vi "Autonomous Independent.vi"() -> ()   [LabVIEW 2014]
doc: "This VI is called when autonomous begins, and will automatically be terminated when autonomous ends. You can carry out timed or sensor driven robot movement independently without needing to return to the caller."
uses:
  <vilib>/Rock Robotics/WPI/Joystick/WPI_JoystickGetSetRefNum.vi
  Support Files/Global Data!!!.vi
panel:
  out "Current State":string
  in  "Recycling Conainer?":bool
  in  "Totes Collected":i8(knob) scale=0.0..3.0
  in  "Direction?":bool
  # "Be sure to right-click and choose Data Operations>>Make Current Value default if you want to save the array values with the VI"
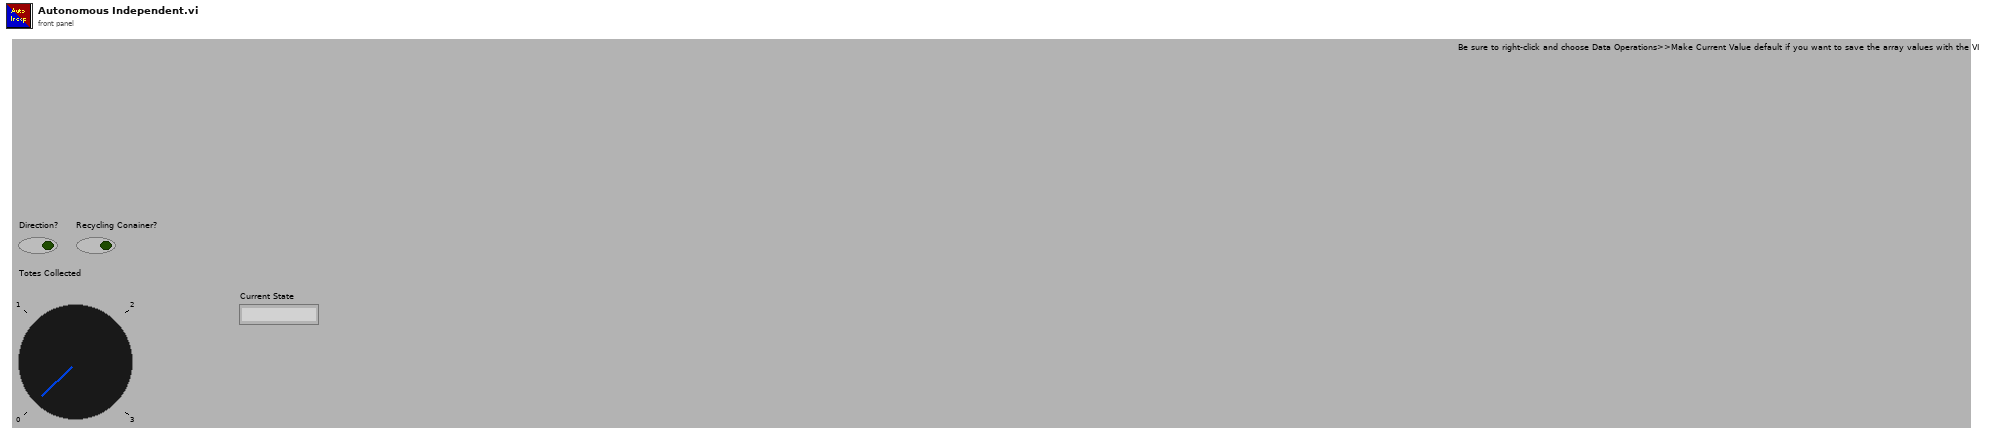
[diagram p1: front panel]
types:
  T1 = typedef "WPI_JoystickDevRef.ctl" = cluster{"Device":T2}
  T2 = typedef "WPI_JoystickDeviceEnum.ctl" = enum16{"USB 0", "USB 1", "USB 2", "USB 3", "USB 4", "USB 5"}
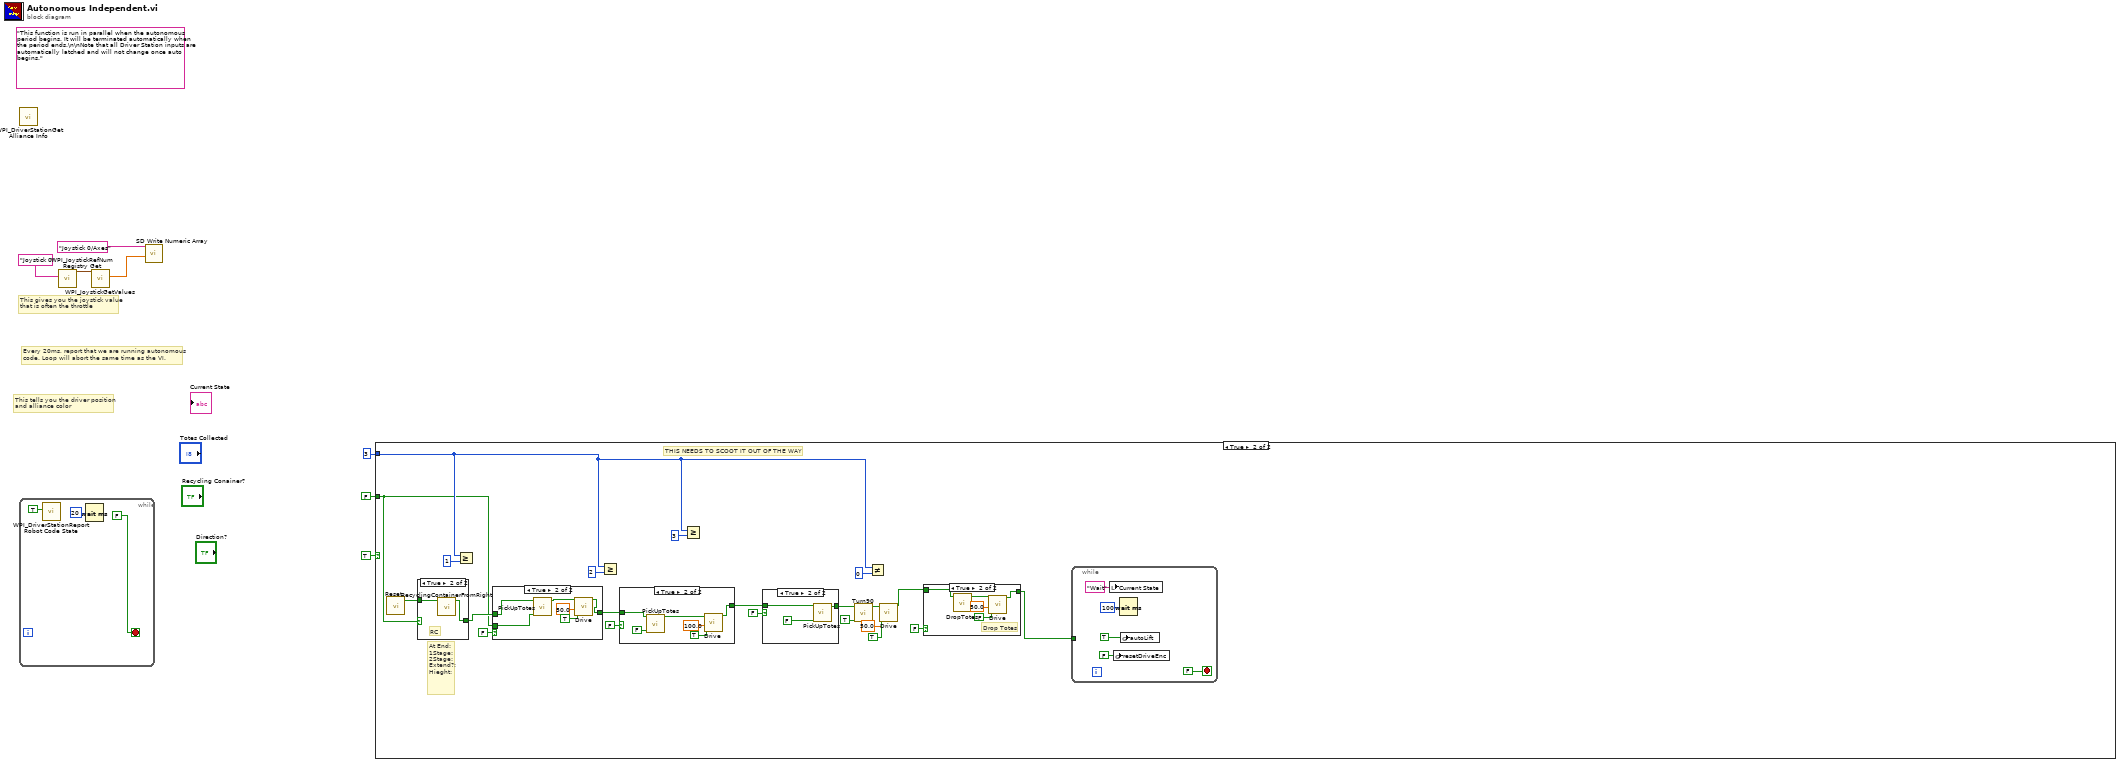
[diagram p0: block diagram]
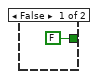
[diagram p3: hidden frame]
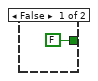
[diagram p4: hidden frame]
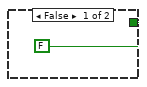
[diagram p5: hidden frame]
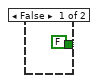
[diagram p6: hidden frame]
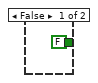
[diagram p7: hidden frame]
diagram:
  (unwired) "This function is run in parallel when the autonomous period begins. It will be terminated automatically when the period ends.\n\nNote that all Driver Station inputs are automatically latched and will not change once auto begins."
  # "Every 20ms, report that we are running autonomous\ncode. Loop will abort the same time as the VI."
  # "This gives you the joystick value\nthat is often the throttle"
  # "This tells you the driver position\nand alliance color"
  n1 = while {
    stop <- FALSE stop-if-true
    n2 = call <vilib>:"WPI_DriverStationReport Robot Code State.vi"("Autonomous"=TRUE) -> ()  [unwired: 10 in, 1 out]
    n3 = Wait (ms)(milliseconds to wait=u32 20) -> ()  [unwired: 1 out]
  }
  n4 = call <vilib>:"WPI_DriverStationGet Alliance Info.vi"() -> ()  [unwired: 12 out]
  n5 = call <vilib>:"WPI_JoystickRefNum Registry Get.vi"("refnum name"="Joystick 0") -> ("JoystickDevRef"=w6:T1)  [unwired: 1 in, 9 out]
  n6 = call <vilib>:"WPI_JoystickGetValues.vi"("JoystickDevRef"=w6) -> ("Axes"=w4:dbl[])  [unwired: 6 in, 4 out]
  n7 = call <vilib>:"SD Write Numeric Array.vi"("Numeric Array"=w4, "Name"="Joystick 0/Axes") -> ()  [unwired: 8 in, 2 out]
  n8 = case shown="True" TRUE {
    tunnel: i8 3 ("Totes Collected") -> [_ w27]
    tunnel: FALSE ("Recycling Conainer?") -> [_ w23]
    frame False {
    }
    frame True {
      # "At End:\n1Stage:\n2Stage:\nExtend?:\nHieght:"
      # "THIS NEEDS TO SCOOT IT OUT OF THE WAY"
      n9 = call "Reset.vi"() -> ("Boolean"=w24:bool)  [unwired: 11 in]
      n10 = case shown="True" w23 {
        tunnel: [FALSE w63] -> w31
        tunnel: w24 -> [_ w62]
        frame False {
        }
        frame True {
          # "RC"
          n11 = call "RecyclingContainerFromRight.vi"("Boolean In"=w62) -> ("Boolean Out"=w63:bool)  [unwired: 9 in]
        }
      }
      n12 = Greater Or Equal?(x=w27, y=i8 1) -> ()  [unwired: 1 out]
      n13 = case shown="True" FALSE {
        tunnel: w31 -> [_ w58]
        tunnel: [FALSE w59] -> w22
        tunnel: w23 -> [_ w57]
        frame False {
        }
        frame True {
          n14 = call "PickUpTotes.vi"("RC?"=w57, "Boolean Out"=w58) -> ("Boolean"=w60:bool)  [unwired: 9 in]
          n15 = call "Drive.vi"("Backward?"=TRUE, "Distance"=50.0, "Boolean in"=w60) -> ("Boolean out"=w59:bool)  [unwired: 8 in]
        }
      }
      n16 = Greater Or Equal?(x=w27, y=i8 2) -> ()  [unwired: 1 out]
      n17 = case shown="True" FALSE {
        tunnel: w22 -> [_ w41]
        tunnel: [FALSE ("Boolean out") w39] -> w21
        frame False {
        }
        frame True {
          n18 = call "PickUpTotes.vi"("RC?"=FALSE, "Boolean Out"=w41) -> ("Boolean"=w42:bool)  [unwired: 9 in]
          n19 = call "Drive.vi"("Backward?"=TRUE, "Distance"=100.0, "Boolean in"=w42) -> ("Boolean out"=w39:bool)  [unwired: 8 in]
        }
      }
      n20 = Greater Or Equal?(x=w27, y=i8 3) -> ()  [unwired: 1 out]
      n21 = case shown="True" FALSE {
        tunnel: w21 -> [_ w34]
        tunnel: [FALSE ("Boolean") w33] -> w20
        frame False {
        }
        frame True {
          n22 = call "PickUpTotes.vi"("RC?"=FALSE, "Boolean Out"=w34) -> ("Boolean"=w33:bool)  [unwired: 9 in]
        }
      }
      n23 = call "Turn90.vi"("Right?"=TRUE, "Boolean in"=w20) -> ("Boolean out"=w18:bool)  [unwired: 9 in]
      n24 = Not Equal?(x=w27, y=i8 0) -> ()  [unwired: 1 out]
      n25 = call "Drive.vi"("Backward?"=TRUE, "Distance"=50.0, "Boolean in"=w18) -> ("Boolean out"=w16:bool)  [unwired: 8 in]
      n26 = case shown="True" FALSE {
        tunnel: [FALSE w51] -> w25
        tunnel: w16 -> [_ w53]
        frame False {
        }
        frame True {
          # "Drop Totes"
          n27 = call "DropTotes.vi"("Boolean In"=w53) -> ("Boolean Out"=w52:bool)  [unwired: 10 in]
          n28 = call "Drive.vi"("Backward?"=FALSE, "Distance"=50.0, "Boolean in"=w52) -> ("Boolean out"=w51:bool)  [unwired: 8 in]
        }
      }
      n29 = while {
        tunnel: w25 -> [_]
        stop <- FALSE stop-if-true
        n30 = local write "Current State"("Wait" ("Current State")) -> ()
        n31 = global write "Global Data!!!.vi" "resetDriveEnc"(FALSE ("resetDriveEnc")) -> ()
        n32 = Wait (ms)(milliseconds to wait=u32 100) -> ()  [unwired: 1 out]
        n33 = global write "Global Data!!!.vi" "autoLift"(TRUE ("resetDriveEnc")) -> ()
      }
    }
  }
